vi "Patrick-multichannel-Sim-Aq.vi"(4 "Cluster":T1={"1/f vs. Uniform "=1.0, "DC Drift Fraction"=0.0, "DC Drift Freq"=0.19999999999999996, "DC Offset"=0.0, "60Hz Amplitude"=0.005, "Gauss/Unif %"=0.5, "Sig Amp"=1.0, "Noise Amp"=0.005} {"Noise Amp" format="%.1p"; "Sig Amp" format="%.2p"; "Gauss/Unif %" min=0.0 max=1.0 step=0.05 format="%.2f"; "60Hz Amplitude" min=0.0 max=10.0 step=0.05 format="%.2p"; "DC Offset" min=-1.0 max=1.0 step=0.01 format="%.2f"; "DC Drift Freq" min=0.0 max=5.0 step=0.05 format="%.2f"; "DC Drift Fraction" format="%.2f"; "1/f vs. Uniform" min=0.0 max=50.0 step=0.5 format="%.1p"}, 5 "data":waveform(dbl)[](array[waveform]), 6 "sampling info":cluster{"Fs":dbl, "#s":dbl}={"Fs"=204800.0, "#s"=20480.0}) -> (0 "Data":waveform(dbl)[](array[waveform])=[{"t0"=timestamp(0 s since 1904-01-01), "dt"=4.8828125e-06, "Y"=array[20480 elements]}, {"t0"=timestamp(0 s since 1904-01-01), "dt"=4.8828125e-06, "Y"=array[20480 elements]}, {"t0"=timestamp(0 s since 1904-01-01), "dt"=4.8828125e-06, "Y"=array[20480 elements]}, {"t0"=timestamp(0 s since 1904-01-01), "dt"=4.8828125e-06, "Y"=array[20480 elements]}, {"t0"=timestamp(0 s since 1904-01-01), "dt"=4.8828125e-06, "Y"=array[20480 elements]}, {"t0"=timestamp(0 s since 1904-01-01), "dt"=4.8828125e-06, "Y"=array[20480 elements]}, {"t0"=timestamp(0 s since 1904-01-01), "dt"=4.8828125e-06, "Y"=array[20480 elements]}, {"t0"=timestamp(0 s since 1904-01-01), "dt"=4.8828125e-06, "Y"=array[20480 elements]}])   [LabVIEW 2013]
uses:
  <vilib>/Analysis/2dsp.llb/Real FFT.vi
  <vilib>/Analysis/2dsp.llb/Inverse Real FFT.vi
  <vilib>/Analysis/2dsp.llb/Decimate (single shot).vi
  <vilib>/Analysis/2dsp.llb/Decimate (single shot, DBL).vi
  <vilib>/Analysis/3filter.llb/Butterworth Filter (DBL).vi
  <vilib>/Utility/error.llb/Error Cluster From Error Code.vi
  <vilib>/measure/NI_MABase.lvlib
  <vilib>/Analysis/NI_AALPro.lvlib
  <vilib>/Analysis/NI_AALBase.lvlib
panel:
  out "Waveform Graph":waveform(dbl)[](graph)=[{"t0"=timestamp(0 s since 1904-01-01), "dt"=4.8828125e-06, "Y"=array[20480 elements]}, {"t0"=timestamp(0 s since 1904-01-01), "dt"=4.8828125e-06, "Y"=array[20480 elements]}, {"t0"=timestamp(0 s since 1904-01-01), "dt"=4.8828125e-06, "Y"=array[20480 elements]}, {"t0"=timestamp(0 s since 1904-01-01), "dt"=4.8828125e-06, "Y"=array[20480 elements]}, {"t0"=timestamp(0 s since 1904-01-01), "dt"=4.8828125e-06, "Y"=array[20480 elements]}, {"t0"=timestamp(0 s since 1904-01-01), "dt"=4.8828125e-06, "Y"=array[20480 elements]}, {"t0"=timestamp(0 s since 1904-01-01), "dt"=4.8828125e-06, "Y"=array[20480 elements]}, {"t0"=timestamp(0 s since 1904-01-01), "dt"=4.8828125e-06, "Y"=array[20480 elements]}]
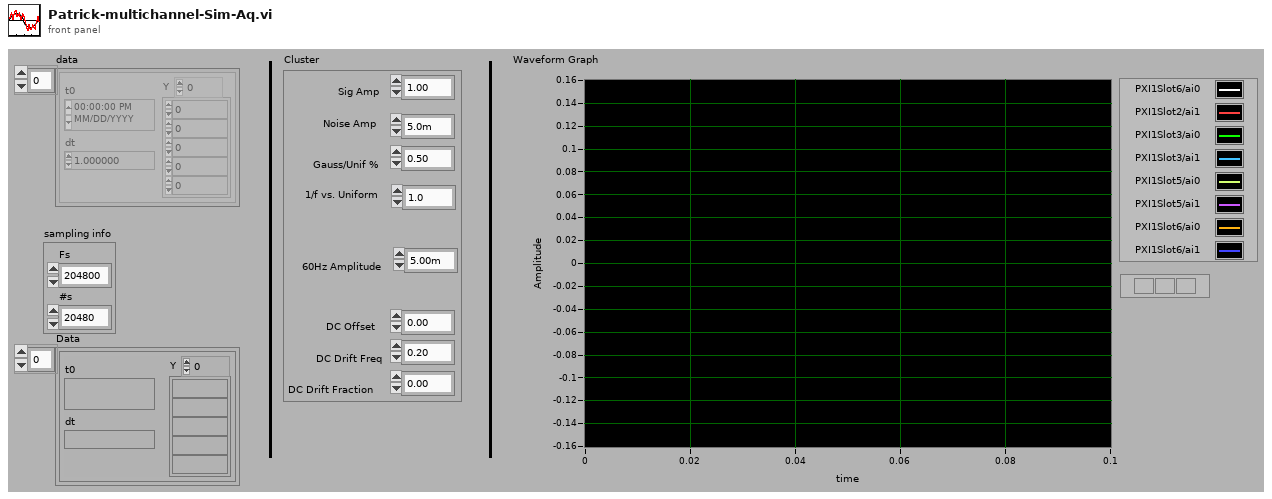
[diagram p1: front panel]
types:
  T1 = cluster{"1/f vs. Uniform ":dbl, "DC Drift Fraction":dbl, "DC Drift Freq":dbl, "DC Offset":dbl, "60Hz Amplitude":dbl, "Gauss/Unif %":dbl, "Sig Amp":dbl, "Noise Amp":dbl}
  T2 = enum32{"Lowpass", "Highpass", "Bandpass", "Bandstop"}
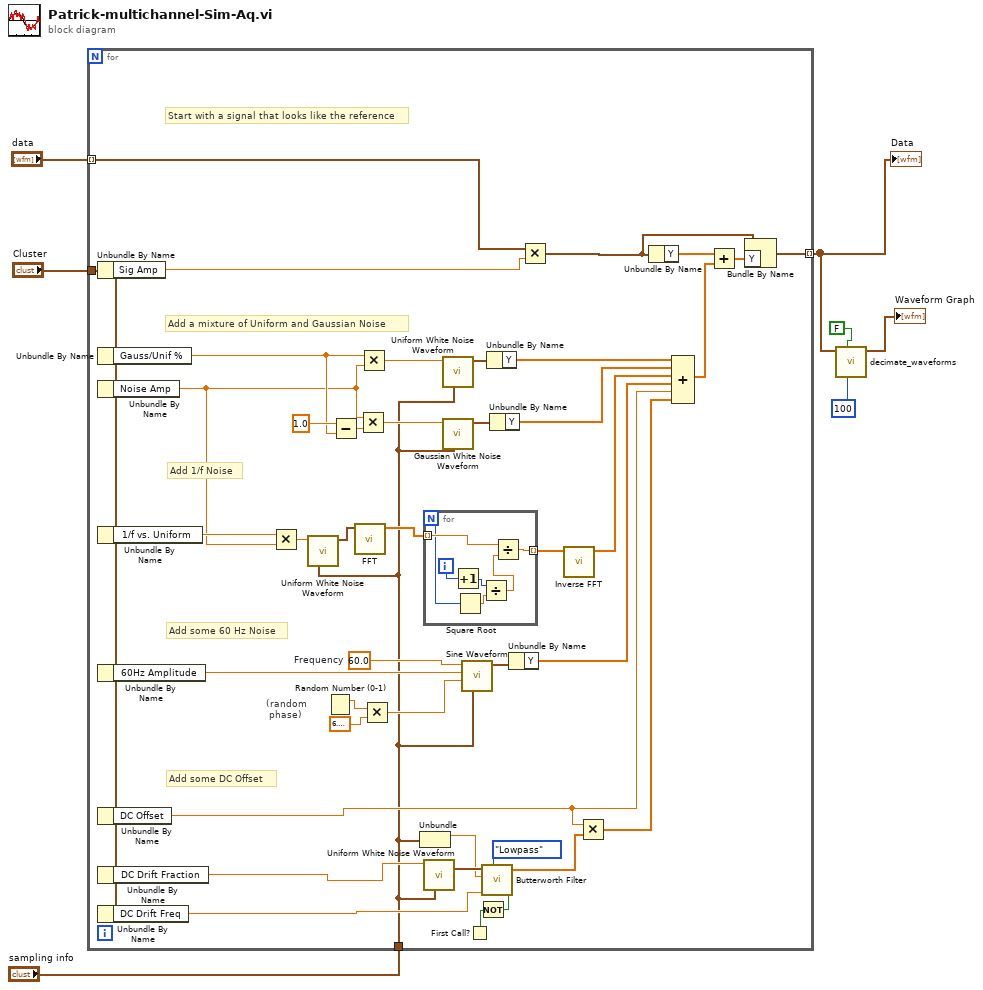
[diagram p0: block diagram]
diagram:
  n1 = for {
    tunnel: "Cluster" -> [w17]
    tunnel: "sampling info" -> [w14]
    tunnel: "data" -> [w12] mode=indexing
    tunnel: [w8] -> w3 mode=indexing
    w43 = 60.0  # Frequency
    # "Start with a signal that looks like the reference"
    # "Add 1/f Noise"
    # "(random\n phase)"
    # "Add some DC Offset"
    # "Add some 60 Hz Noise"
    # "Add a mixture of Uniform and Gaussian Noise"
    n2 = Unbundle By Name(w17) -> ("Sig Amp"=w13:dbl)
    n3 = Unbundle By Name(w17) -> ("Gauss/Unif %"=w22:dbl)
    n4 = Unbundle By Name(w17) -> ("Noise Amp"=w20:dbl)
    n5 = Unbundle By Name(w17) -> ("1/f vs. Uniform"=w21:dbl)
    n6 = Unbundle By Name(w17) -> ("60Hz Amplitude"=w19:dbl)
    n7 = Unbundle By Name(w17) -> ("DC Offset"=w18:dbl)
    n8 = Unbundle By Name(w17) -> ("DC Drift Fraction"=w15:dbl)
    n9 = Unbundle By Name(w17) -> ("DC Drift Freq"=w16:dbl)
    n10 = Multiply(x=w21, y=w20) -> (x*y=w30:dbl)
    n11 = call <vilib>:"Uniform White Noise Waveform.vi"("sampling info"=w14, "amplitude"=w30) -> ("signal out"=w29:waveform(dbl))  [unwired: 8 in, 1 out]
    n12 = Random Number (0-1)() -> (number: 0 to 1=w41:dbl)
    n13 = Subtract(x=1.0, y=w22) -> (x-y=w45:dbl)
    n14 = call-poly <vilib>:"FFT.vi"("X"=w29) -> ("FFT {X}"=w32:cdb[])  [unwired: 9 in, 1 out]
    n15 = Multiply(x=w20, y=w45) -> (x*y=w47:dbl)
    n16 = Multiply(x=w22, y=w20) -> (x*y=w46:dbl)
    n17 = Multiply(x=w41, y=6.283185307179586) -> (x*y=w40:dbl)
    n18 = Unbundle(w14) -> ("Fs"=w37:dbl)  [unwired: 1 out]
    n19 = for {
      N -> [w53]
      tunnel: [w56] -> w31 mode=indexing
      tunnel: w32 -> [w55] mode=indexing
      i -> [w54]
      n20 = Increment(x=w54) -> (x+1=w51:i32)
      n21 = Square Root(x=w53) -> (sqrt(x)=w52:dbl)
      n22 = Divide(x=w51, y=w52) -> (x/y=w50:dbl)
      n23 = Divide(x=w55, y=w50) -> (x/y=w56:cdb)
    }
    n24 = call <vilib>:"Uniform White Noise Waveform.vi"("sampling info"=w14, "amplitude"=w15) -> ("signal out"=w38:waveform(dbl))  [unwired: 8 in, 1 out]
    n25 = call <vilib>:"Uniform White Noise Waveform.vi"("sampling info"=w14, "amplitude"=w46) -> ("signal out"=w48:waveform(dbl))  [unwired: 8 in, 1 out]
    n26 = call <vilib>:"Gaussian White Noise Waveform.vi"("sampling info"=w14, "standard deviation"=w47) -> ("signal out"=w49:waveform(dbl))  [unwired: 8 in, 1 out]
    n27 = call <vilib>:"Sine Waveform.vi"("sampling info"=w14, "phase"=w40, "amplitude"=w19, "frequency"=w43) -> ("signal out"=w39:waveform(dbl))  [unwired: 6 in, 1 out]
    n28 = First Call?() -> (First Call?: T/F=w23:bool)
    n29 = Not(x=w23) -> (.not. x?=w35:bool)
    n30 = call-poly <vilib>:"Butterworth Filter.vi"("init/cont (init:F)"=w35, "filter type"=T2."Lowpass", "low cutoff freq: fl"=w16, "sampling freq: fs"=w37, "X"=w38) -> ("Filtered X"=w34:dbl[])  [unwired: 3 in, 1 out]
    n31 = Unbundle By Name(w48) -> ("Y"=w33:dbl[])
    n32 = Unbundle By Name(w49) -> ("Y"=w24:dbl[])
    n33 = Unbundle By Name(w39) -> ("Y"=w28:dbl[])
    n34 = Multiply(x=w12, y=w13) -> (x*y=w9:waveform(dbl))
    n35 = call-poly <vilib>:"Inverse FFT.vi"("FFT {X}"=w31) -> ("X"=w27:dbl[])  [unwired: 9 in, 1 out]
    n36 = Multiply(x=w18, y=w34) -> (x*y=w26:dbl[])
    n37 = Unbundle By Name(w9) -> ("Y"=w11:dbl[])
    n38 = Compound Arithmetic op=ADD(w33, w24, w27, w28, w18, w26) -> (w25:dbl[])
    n39 = Add(x=w11, y=w25) -> (x+y=w10:dbl[])
    n40 = Bundle By Name(cluster=w9, "Y"=w10) -> (w8:waveform(dbl))
  }
  "Data" <- w3
  n41 = call "decimate_waveforms.vi"("decimating factor"=100, "averaging"=FALSE, "Input Signal"=w3) -> ("Decimated Waveforms"=→"Waveform Graph":waveform(dbl)[])  [unwired: 7 in, 1 out]
